vi "QCA - DUT Abort RX.vi"(0 "CART TCP Connection In":refnum<k5>, 11 "error in (no error)":errorcluster, 12 "Read Time Out(ms)":i32=10) -> (4 "CART TCP Connection Out":refnum<k5>, 10 "TX Response":T1, 15 "error out":errorcluster)   [LabVIEW 2012]
uses:
  Controls/Parameter.ctl
  Controls/QCA NART Response Type.ctl
  Controls/QCA NART Response SubType.ctl
panel:
  out "error out 2":errorcluster
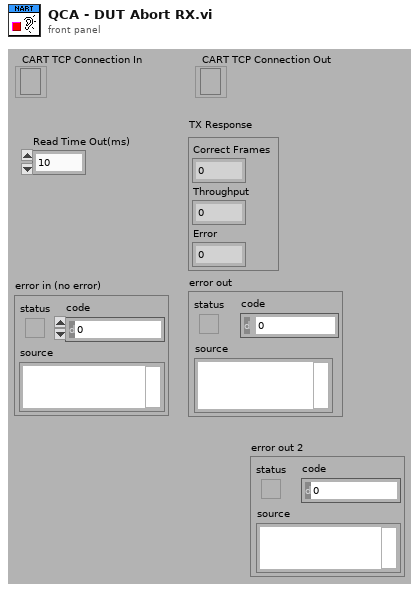
[diagram p1: front panel]
types:
  T1 = cluster{"Correct Frames":i32, "Throughput":i32, "Error":i32}
  T2 = typedef "QCA NART Response SubType.ctl" = enum16{"NONE", "OK", "ON", "OFF", "BEGIN", "DONE"}
  T3 = typedef "Parameter.ctl" = cluster{"Name":string, "Type":enum16{"decimal", "string", "float", "hex"}}
  T4 = typedef "QCA NART Response Type.ctl" = enum16{"DEBUG", "CONTROL", "INFO", "WARNING", "ERROR", "NONE"}
  T5 = typedef "QCA NART Message.ctl" = cluster{"Code":dbl, "Response Type":T4, "Response Subtype":T2, "Message":string}
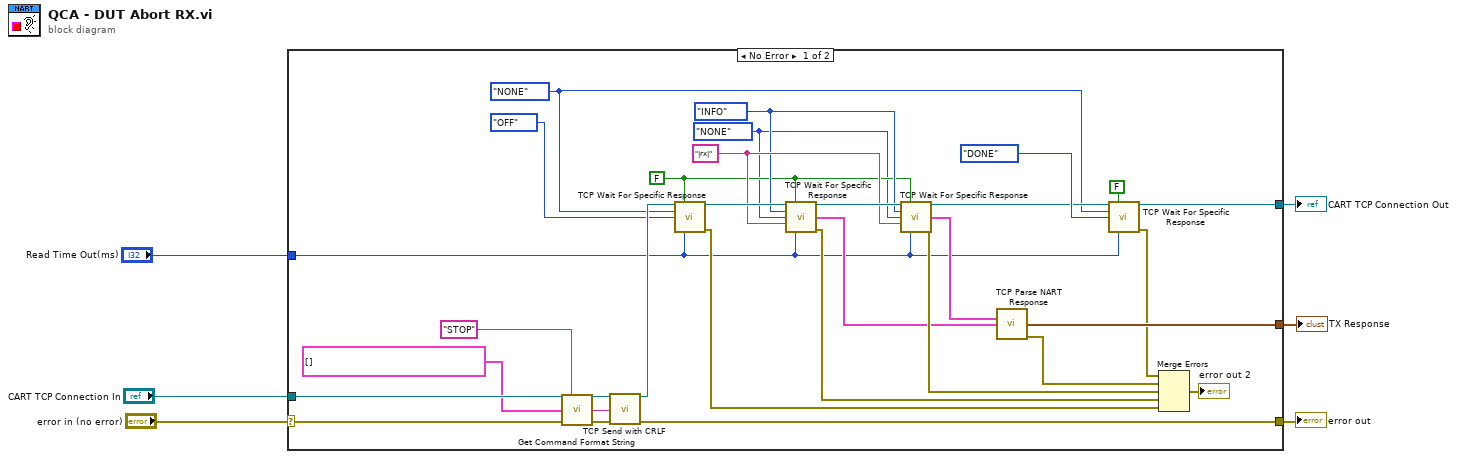
[diagram p0: block diagram]
diagram:
  n1 = case shown="No Error" "error in (no error)" {
    selector: "error in (no error)" -> [w31 w37]
    tunnel: [w28 w37] -> w5
    tunnel: "CART TCP Connection In" -> [w35 w36]
    tunnel: [w29 w36] -> w3
    tunnel: [w27 _] -> w2
    tunnel: "Read Time Out(ms)" -> [w7 _]
    frame No Error {
      w8 = QCA_NART_Response_SubType."NONE" ("Response Subtype")
      w9 = FALSE ("Next response (t)")
      w14 = QCA_NART_Response_Type."INFO" ("Expected Type")
      w22 = "|rx|" ("Expected Message Start (\"\":any)")
      w13 = QCA_NART_Response_Type."NONE" ("Expected Response")
      n2 = call "Get Command Format String.vi"("Command"="STOP", "Parameters"=T3[] []) -> ("Command Format String"=w32:string)  [unwired: 13 in]
      n3 = call "TCP Send with CRLF.vi"("CART TCP Connection"=w35, "data in"=w32, "error IO"=w31) -> ("CART TCP Connection Out"=w30:refnum<k5>, "error out"=w28:errorcluster)  [unwired: 11 in]
      n4 = call "TCP Wait For Specific Response.vi"("TCP Connection In"=w30, "Next response (t)"=w9, "Expected Type"=w13, "Expected Subtype (none)"=QCA_NART_Response_SubType."OFF" ("Response Subtype"), "Timeout (250 ms)"=w7) -> ("TCP Connection Out"=w24:refnum<k5>, "error out"=w17:errorcluster)  [unwired: 7 in, 2 out]
      n5 = call "TCP Wait For Specific Response.vi"("TCP Connection In"=w24, "Next response (t)"=w9, "Expected Type"=w14, "Expected Subtype (none)"=w8, "Expected Message Start (\"\":any)"=w22, "Timeout (250 ms)"=w7) -> ("TCP Connection Out"=w25:refnum<k5>, "Desired Response"=w11:T5, "error out"=w18:errorcluster)  [unwired: 6 in, 1 out]
      n6 = call "TCP Wait For Specific Response.vi"("TCP Connection In"=w25, "Next response (t)"=w9, "Expected Type"=w14, "Expected Subtype (none)"=w8, "Expected Message Start (\"\":any)"=w22, "Timeout (250 ms)"=w7) -> ("TCP Connection Out"=w23:refnum<k5>, "Desired Response"=w12:T5, "error out"=w19:errorcluster)  [unwired: 6 in, 1 out]
      n7 = call "TCP Parse NART Response.vi"("Response"=w12, "Response Template"=w11) -> ("TX Response"=w27:T1, "error out"=w20:errorcluster)  [unwired: 12 in]
      n8 = call "TCP Wait For Specific Response.vi"("TCP Connection In"=w23, "Next response (t)"=FALSE, "Expected Type"=w13, "Expected Subtype (none)"=QCA_NART_Response_SubType."DONE" ("Response Subtype"), "Timeout (250 ms)"=w7) -> ("TCP Connection Out"=w29:refnum<k5>, "error out"=w21:errorcluster)  [unwired: 7 in, 2 out]
      n9 = Merge Errors(w21, w20, w19, w18, w17) -> (→"error out 2":errorcluster)
    }
    frame Error {
    }
  }
  "error out" <- w5
  "CART TCP Connection Out" <- w3
  "TX Response" <- w2
